vi "tio32_WriteDac.vi"(0 "VISA resource name":refnum<visa-resource-name>, 5 "Board address":i32=4660 format="%x", 7 "DAC number":i32=1, 9 "mode":i32=1, 11 "error in (no error)":errorcluster, 12 "value":dbl=666.0, 13 "User Ref":dbl=2.5) -> (4 "VISA resource name out":refnum<visa-resource-name>, 6 "return":i32=666, 15 "error out":errorcluster)   [LabVIEW 2011]
uses:
  l_pse_dll/Tio32.dll
panel:
  # "tio32_WriteDac"
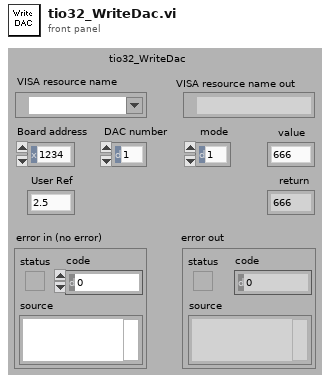
[diagram p1: front panel]
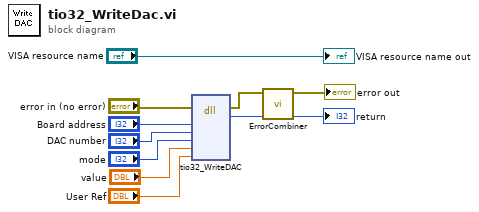
[diagram p0: block diagram]
diagram:
  n1 = dll-call lib="C:/Users/Ikaika's/Documents/DCC/Apps/INA231/INA231-SFT-rev1/INA231-Sourcecode-rev1/INA231/Shell Resources/l_pse_dll/Tio32.dll" fn="tio32_WriteDAC" label="tio32_WriteDac()"(error in="error in (no error)", "adr"="Board address", "dacNo"="DAC number", "dacMode"="mode", "val"="value", "refUser"="User Ref") -> (error out=w6:errorcluster, "Rückgabetyp"=w7:i32)  [unwired: 7 in, 1 out]
  n2 = call "ErrorCombiner.vi"("Return In"=w7, "error in (no error)"=w6) -> ("Return Out"=→"return":i32, "error out"=→"error out":errorcluster)  [unwired: 8 in]
  "VISA resource name out" <- "VISA resource name"
